vi "Update Title.vi"(8 "error in (no error)":errorcluster, 10 "Title":T1={"Enable"=FALSE, "Title"="", "Docking"=0, "Over Plot?"=FALSE, "Font"={"Name"="", "Size"=0.0, "style"=0, "Color"={"Color"=0, "alpha"=76}}, "Background"={"Color"={"Color"=0, "alpha"=76}, "HatchStyle"=0, "GradientStyle"=0}, "Border"={"color"={"Color"=0, "alpha"=76}, "DashStyle"=enum."Solid", "Width"=2}} {"Border"."color"."alpha" scale=0.0..255.0; "Background"."GradientStyle" items=["None", "LeftRight", "TopBottom", "Center", "DiagonalLeft", "DiagonalRight", "HorizontalCenter", "VerticalCenter"]; "Background"."HatchStyle" items=["None", "BackwardDiagonal", "Cross", "DarkDownwardDiagonal", "DarkHorizontal", "DarkUpwardDiagonal", "DarkVertical", "DashedDownwardDiagonal", "DashedHorizontal", "DashedUpwardDiagonal", "DashedVertical", "DiagonalBrick", "DiagonalCross", "Divot", "DottedDiamond", "DottedGrid", "ForwardDiagonal", "Horizontal", "HorizontalBrick", "LargeCheckerBoard", "LargeConfetti", "LargeGrid", "LightDownwardDiagonal", "LightHorizontal", "LightUpwardDiagonal", "LightVertical", "NarrowHorizontal", "NarrowVertical", "OutlinedDiamond", "Percent05", "Percent10", "Percent20", "Percent25", "Percent30", "Percent40", "Percent50", "Percent60", "Percent70", "Percent75", "Percent80", "Percent90", "Plaid", "Shingle", "SmallCheckerBoard", "SmallConfetti", "SmallGrid", "SolidDiamond", "Sphere", "Trellis", "Vertical", "Wave", "Weave", "WideDownwardDiagonal", "WideUpwardDiagonal", "ZigZag"]; "Background"."Color"."alpha" scale=0.0..255.0; "Font"."Color"."alpha" scale=0.0..255.0; "Font"."style" items=["Regular"=0, "Bold"=1, "Italic"=2, "Underline"=4, "Strikeout"=8]; "Font"."Size" min=4.0 max=100.0; "Docking" items=["Top", "Right", "Bottom", "Left", "None"]}, 11 ".NET Refnum in":refnum<k24>) -> (0 "error out":errorcluster, 3 ".NET Refnum out":refnum<k24>)   [LabVIEW 2014, in "XMSChart.xctl"]
uses:
  XMSChart.xctl
  System.Windows.Forms.DataVisualization
  Controls/Title.ctl
  Controls/Font.ctl
  Controls/Color.ctl
  Controls/Background.ctl
  Controls/Border.ctl
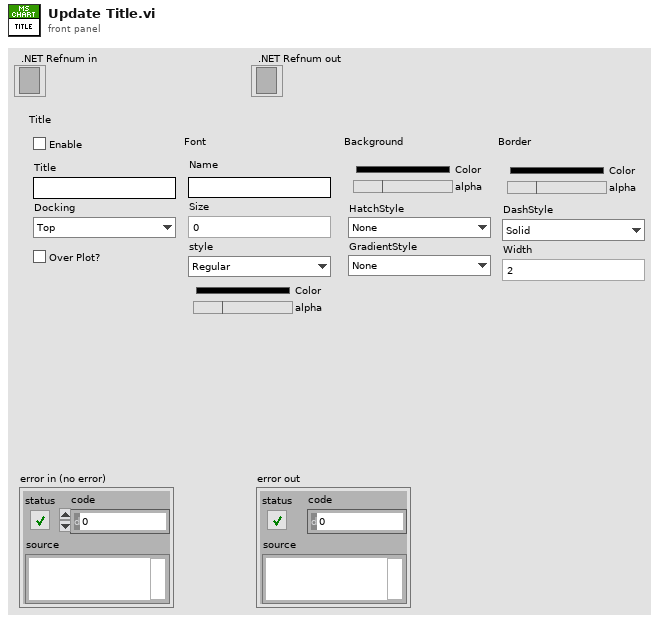
[diagram p1: front panel]
types:
  T1 = typedef "XMSChart.xctl/Title.ctl" = cluster{"Enable":bool, "Title":string, "Docking":i32, "Over Plot?":bool, "Font":T2, "Background":T4, "Border":T5}
  T2 = typedef "XMSChart.xctl/Font.ctl" = cluster{"Name":string, "Size":dbl, "style":i32, "Color":T3}
  T3 = typedef "XMSChart.xctl/Color.ctl" = cluster{"Color":u32, "alpha":u8}
  T4 = typedef "XMSChart.xctl/Background.ctl" = cluster{"Color":T3, "HatchStyle":i32, "GradientStyle":i32}
  T5 = typedef "XMSChart.xctl/Border.ctl" = cluster{"color":T3, "DashStyle":enum16{"NotSet", "Dash", "DashDot", "DashDotDot", "Dot", "Solid"}, "Width":i32}
  T6 = enum16{"NotSet", "Dash", "DashDot", "DashDotDot", "Dot", "Solid"}
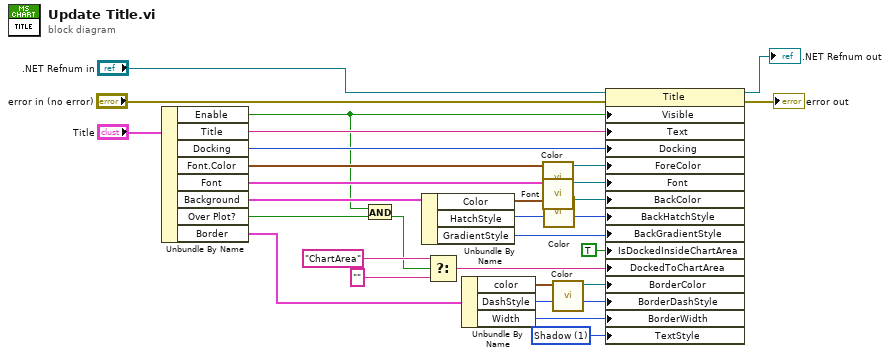
[diagram p0: block diagram]
diagram:
  w1 = 1 items=["Default", "Shadow", "Emboss", "Embed", "Frame"] ("TextStyle")
  n1 = Unbundle By Name("Title") -> ("Enable"=w7:bool, "Title"=w20:string, "Docking"=w19:i32, "Font.Color"=w21:T3, "Font"=w27:T2, "Background"=w18:T4, "Over Plot?"=w10:bool, "Border"=w6:T5)
  n2 = And(x=w7, y=w10) -> (x .and. y?=w8:bool)
  n3 = Unbundle By Name(w18) -> ("Color"=w17:T3, "HatchStyle"=w15:i32, "GradientStyle"=w14:i32)
  n4 = Select(t="ChartArea" ("DockedToChartArea"), s=w8, f="") -> (s? t:f=w9:string)
  n5 = Unbundle By Name(w6) -> ("color"=w5:T3, "DashStyle"=w3:T6, "Width"=w2:i32)
  n6 = call "Color.vi"("BGK Color"=w21) -> (".NET Refnum out"=w26:refnum<k24>)  [unwired: 10 in]
  n7 = call "Font.vi"("font"=w27) -> (".NET MSChart Font"=w28:refnum<k24>)  [unwired: 10 in]
  n8 = call "Color.vi"("BGK Color"=w17) -> (".NET Refnum out"=w16:refnum<k24>)  [unwired: 10 in]
  n9 = call "Color.vi"("BGK Color"=w5) -> (".NET Refnum out"=w4:refnum<k24>)  [unwired: 10 in]
  n10 = property on="Property Node" class="Title"(reference=".NET Refnum in", error in="error in (no error)", "Visible"=w7, "Text"=w20, "Docking"=w19, "ForeColor"=w26, "Font"=w28, "BackColor"=w16, "BackHatchStyle"=w15, "BackGradientStyle"=w14, "IsDockedInsideChartArea"=TRUE, "DockedToChartArea"=w9, "BorderColor"=w4, "BorderDashStyle"=w3, "BorderWidth"=w2, "TextStyle"=w1) -> (reference out=→".NET Refnum out":refnum<k24>, error out=→"error out":errorcluster)
